vi "DSDLL Close Virtual Channels.vi"(8 "error in":errorcluster, 11 "dsdll in":T1) -> (0 "error out":errorcluster, 3 "dsdll out":T1)   [LabVIEW 2018, in "DSDLL Virtual Digitizer.lvlib"]
doc: "Close all virtual channels. Executes even if error is on the input. Call this after the measurement is done and ADC not needed anymore."
uses:
  DSDLL Virtual Digitizer.lvlib
  DSDLL Session.ctl
  dsdll source distribution/dsdll_instance.ctl
  dsdll source distribution/dsdll_device_record.ctl
  DSDLL Process Config.ctl
  DSDLL Data Packet.ctl
  dsdll source distribution/dsdll.lvlib
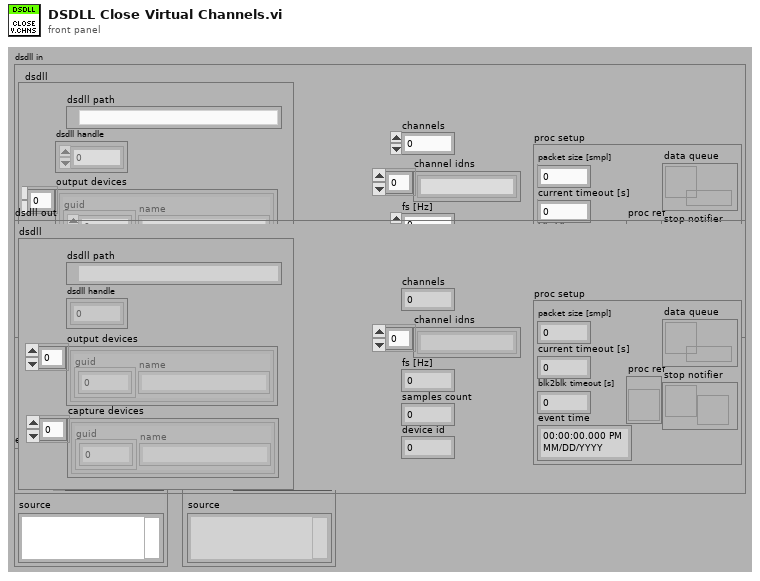
[diagram p1: front panel]
types:
  T1 = typedef "DSDLL Virtual Digitizer.lvlib/DSDLL Session.ctl" = cluster{"dsdll":T2, "channels":i32, "device id":i32, "channel idns":string[], "proc setup":T4, "samples count":i32, "fs [Hz]":dbl}
  T2 = typedef "dsdll.lvlib/dsdll_instance.ctl" = cluster{"dsdll path":path, "dsdll handle":u8[], "output devices":T3[], "capture devices":T3[]}
  T3 = typedef "dsdll.lvlib/dsdll_device_record.ctl" = cluster{"guid":u8[], "name":string}
  T4 = typedef "DSDLL Virtual Digitizer.lvlib/DSDLL Process Config.ctl" = cluster{"packet size [smpl]":i32, "current timeout [s]":dbl, "blk2blk timeout [s]":dbl, "event time":timestamp, "data queue":refnum<queue>, "stop notifier":refnum<notifier>, "proc ref":refnum<vi>}
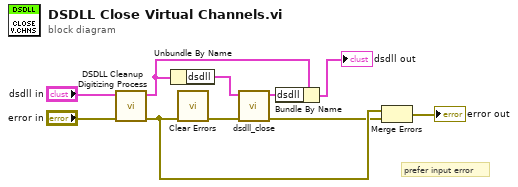
[diagram p0: block diagram]
diagram:
  # "prefer input error"
  n1 = call "DSDLL Cleanup Digitizing Process.vi"("error in"="error in", "dsdll in"="dsdll in") -> ("error out"=w7:errorcluster, "dsdll out"=w3:T1)  [unwired: 8 in]
  n2 = Unbundle By Name(w3) -> ("dsdll"=w4:T2)
  n3 = call <vilib>:"Clear Errors.vi"("error in (no error)"=w7) -> ("error out"=w5:errorcluster)  [unwired: 5 in, 1 out]
  n4 = call "dsdll_close.vi"("error in"=w5, "dsdll instance in"=w4) -> ("error out"=w6:errorcluster, "dsdll instance out"=w2:T2)  [unwired: 8 in]
  n5 = Bundle By Name(cluster=w3, "dsdll"=w2) -> (→"dsdll out":T1)
  n6 = Merge Errors(w7, w6) -> (→"error out":errorcluster)
